vi "test Signed and Unsigned.vi"(8 "error in (no error)":errorcluster, 11 "TestCase in":refnum<class "BNR.lvclass">) -> (0 "error out":errorcluster, 3 "TestCase out":refnum<class "BNR.lvclass">)   [LabVIEW 2020, in "BNR.lvclass"]
uses:
  BNR.lvclass
  52a9e853-f441-4a14-a3ae-af5dd9b478de.vi
  fabf7f84-3cd3-4adf-92be-b1484a105bea.vi
  1abdb739-fb66-4f21-b2ba-a9918976e5c4.vi
  65c3b74b-7b29-4765-ab7a-f8a38be437e9.vi
  4bb312ad-4e10-4980-9d7d-1c2267be8d4c.vi
  52a9e853-f441-4a14-a3ae-af5dd9b478de.vi/9377bb8f-44b5-4a8f-87f1-966fd5a9edcc.vi
  fabf7f84-3cd3-4adf-92be-b1484a105bea.vi/9377bb8f-44b5-4a8f-87f1-966fd5a9edcc.vi
  1abdb739-fb66-4f21-b2ba-a9918976e5c4.vi/16a2565b-3c16-407b-a626-9da2a3da432e.vi
  65c3b74b-7b29-4765-ab7a-f8a38be437e9.vi/9377bb8f-44b5-4a8f-87f1-966fd5a9edcc.vi
  4bb312ad-4e10-4980-9d7d-1c2267be8d4c.vi/16a2565b-3c16-407b-a626-9da2a3da432e.vi
  <vilib>/addons/_JKI Toolkits/VI Tester/TestCase.llb/TestCase.lvclass
  C:/Program Files (x86)/National Instruments/LabVIEW 2020/vi.lib/addons/_JKI Toolkits/VI Tester/TestCase.llb/TestCase.lvclass
panel:
  out "BNR encoded value":bool[](array[boolean])
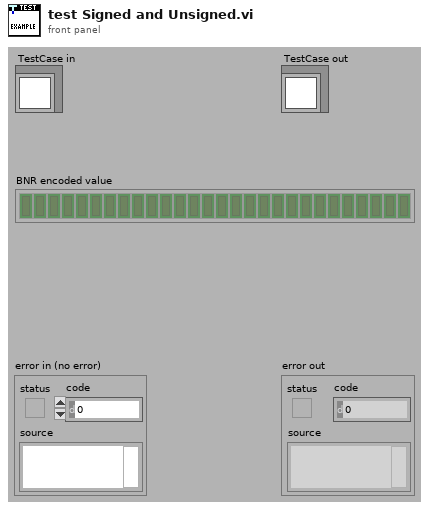
[diagram p1: front panel]
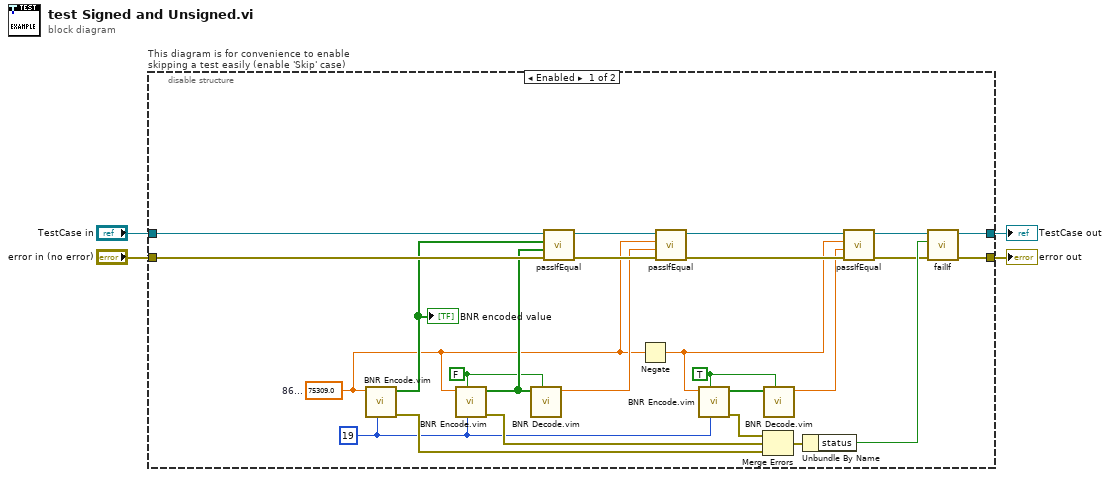
[diagram p0: block diagram]
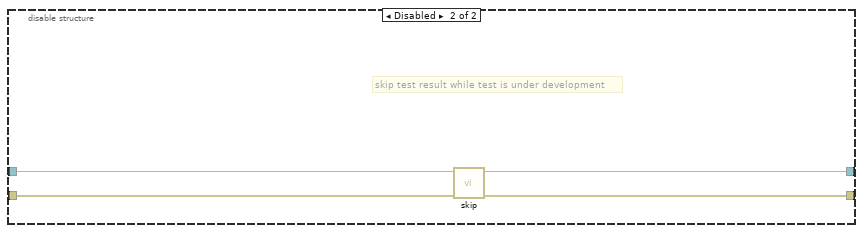
[diagram p2: hidden frame]
diagram:
  n1 = disable-structure "This diagram is for convenience to enable skipping a test easily (enable 'Skip' case)" shown="Enabled" {
    disable-tunnel: "TestCase in" -> [w28 w33]
    disable-tunnel: [w18 w31] -> w2
    disable-tunnel: [w19 w32] -> w1
    disable-tunnel: "error in (no error)" -> [w26 w30]
    frame Enabled {
      w7 = TRUE ("signed")
      w6 = FALSE ("signed")
      w15 = 19 ("data size (bits)")
      w5 = 75309.0  # 86...
      n2 = call "BNR Encode.vim"("data size (bits)"=w15, "value"=w5) -> ("error out"=w17:errorcluster, "BNR encoded value"=w9:bool[])  [unwired: 8 in]
      "BNR encoded value" <- w9
      n3 = call "BNR Encode.vim"("data size (bits)"=w15, "signed"=w6, "value"=w5) -> ("error out"=w16:errorcluster, "BNR encoded value"=w11:bool[])  [unwired: 7 in]
      n4 = call "BNR Decode.vim"("signed"=w6, "BNR encoded value"=w11) -> ("value"=w10:dbl)  [unwired: 9 in]
      n5 = call-dynamic "passIfEqual.vi"("error in (no error)"=w26, "y"=w11, "x"=w9, "TestCase in"=w28) -> ("error out"=w27:errorcluster, "TestCase out"=w29:refnum<class "BNR.lvclass">)  [unwired: 6 in]
      n6 = Negate(x=w5) -> (-x=w8:dbl)
      n7 = call-dynamic "passIfEqual.vi"("error in (no error)"=w27, "y"=w10, "x"=w5, "TestCase in"=w29) -> ("error out"=w25:errorcluster, "TestCase out"=w24:refnum<class "BNR.lvclass">)  [unwired: 6 in]
      n8 = call "BNR Encode.vim"("data size (bits)"=w15, "signed"=w7, "value"=w8) -> ("error out"=w14:errorcluster, "BNR encoded value"=w13:bool[])  [unwired: 7 in]
      n9 = Merge Errors(w14, w16, w17) -> (w23:errorcluster)
      n10 = call "BNR Decode.vim"("signed"=w7, "BNR encoded value"=w13) -> ("value"=w12:dbl)  [unwired: 9 in]
      n11 = Unbundle By Name(w23) -> ("status"=w22:bool)
      n12 = call-dynamic "passIfEqual.vi"("error in (no error)"=w25, "y"=w12, "x"=w8, "TestCase in"=w24) -> ("error out"=w20:errorcluster, "TestCase out"=w21:refnum<class "BNR.lvclass">)  [unwired: 6 in]
      n13 = call-dynamic "failIf.vi"("error in (no error)"=w20, "fail"=w22, "TestCase in"=w21) -> ("error out"=w19:errorcluster, "TestCase out"=w18:refnum<class "BNR.lvclass">)  [unwired: 7 in]
    }
    frame Disabled {
      # "skip test result while test is under development"
      n14 = call <vilib>:"skip.vi"("error in (no error)"=w30, "TestCase in"=w33) -> ("error out"=w32:errorcluster, "TestCase out"=w31:refnum<class "BNR.lvclass">)  [unwired: 8 in]
    }
  }
  "error out" <- w1
  "TestCase out" <- w2
